vi "Move to bounds.vi"(8 "error in (no error)":errorcluster, 9 "Fit parameters":cluster{"Slope":dbl, "Intercept":dbl}, 10 "Seek bounds":cluster{"Minimum":dbl, "Maximum":dbl}, 11 "Motor in":refnum<class "Motor.lvclass">) -> (0 "error out":errorcluster, 2 "Was outside?":bool, 3 "Motor out":refnum<class "Motor.lvclass">)   [LabVIEW 2015, in "Motor.lvclass"]
uses:
  Motor.lvclass
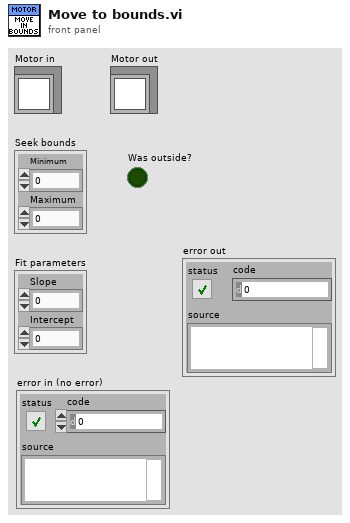
[diagram p1: front panel]
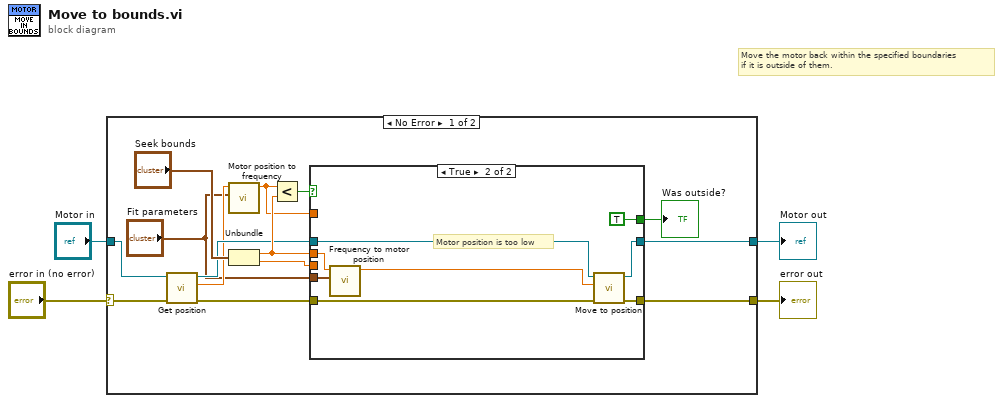
[diagram p0: block diagram]
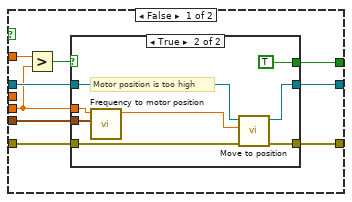
[diagram p2: hidden frame]
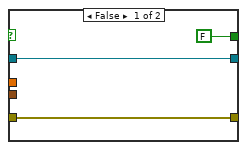
[diagram p3: hidden frame]
diagram:
  # "Move the motor back within the specified boundaries\nif it is outside of them."
  n1 = case shown="No Error" "error in (no error)" {
    selector: "error in (no error)" -> [w9 w48]
    tunnel: [w18 w47] -> w4
    tunnel: [w16 w48] -> w3
    tunnel: "Motor in" -> [w12 w47]
    frame No Error {
      n2 = call-dynamic "Get position.vi"("error in (no error)"=w9, "Motor in"=w12) -> ("error out"=w10:errorcluster, "Position (rev)"=w7:dbl, "Motor out"=w11:refnum<class "Motor.lvclass">)  [unwired: 7 in]
      n3 = call "Motor position to frequency.vi"("Fit parameters"="Fit parameters", "Motor position"=w7) -> ("Frequency"=w6:dbl)  [unwired: 9 in]
      n4 = Unbundle("Seek bounds") -> ("Minimum"=w15:dbl, "Maximum"=w17:dbl)
      n5 = Less?(x=w6, y=w15) -> (x < y?=w14:bool)
      n6 = case shown="True" w14 {
        tunnel: w15 -> [_ w41]
        tunnel: w11 -> [w26 w46]
        tunnel: w10 -> [w25 w45]
        tunnel: [w24 w44] -> w16
        tunnel: w17 -> [w23 _]
        tunnel: [w22 w43] -> w18
        tunnel: [w21 TRUE] -> w8
        tunnel: w6 -> [w20 _]
        tunnel: "Fit parameters" -> [w19 w40]
        frame False {
          n7 = Greater?(x=w20, y=w23) -> (0:w27:bool)
          n8 = case shown="True" w27 {
            tunnel: w26 -> [w29 w38]
            tunnel: w25 -> [w30 w37]
            tunnel: [w30 w36] -> w24
            tunnel: w23 -> [_ w33]
            tunnel: [w29 w35] -> w22
            tunnel: [FALSE TRUE] -> w21
            tunnel: w19 -> [_ w32]
            frame False {
            }
            frame True {
              # "Motor position is too high"
              n9 = call "Frequency to motor position.vi"("Fit parameters"=w32, "Frequency"=w33) -> ("Motor position"=w31:dbl)  [unwired: 9 in]
              n10 = call-dynamic "Move to position.vi"("error in (no error)"=w37, "Position"=w31, "Motor in"=w38) -> ("error out"=w36:errorcluster, "Motor out"=w35:refnum<class "Motor.lvclass">)  [unwired: 7 in]
            }
          }
        }
        frame True {
          # "Motor position is too low"
          n11 = call "Frequency to motor position.vi"("Fit parameters"=w40, "Frequency"=w41) -> ("Motor position"=w39:dbl)  [unwired: 9 in]
          n12 = call-dynamic "Move to position.vi"("error in (no error)"=w45, "Position"=w39, "Motor in"=w46) -> ("error out"=w44:errorcluster, "Motor out"=w43:refnum<class "Motor.lvclass">)  [unwired: 7 in]
        }
      }
      "Was outside?" <- w8
    }
    frame Error {
    }
  }
  "Motor out" <- w4
  "error out" <- w3
